vi "Select Sweep Mode.vi"(8 "error in (no error)":errorcluster, 10 "Sweep Modes":T1, 11 "NRT8000 in":refnum<class "NRT8000.lvclass">) -> (0 "error out":errorcluster, 3 "NRT8000 out":refnum<class "NRT8000.lvclass">)   [LabVIEW 2018, in "NRT8000.lvlib" / "NRT8000.lvclass"]
uses:
  NRT8000.lvclass
  PPLs/Optical Spectrum Analyzer/Parent/OSA.lvlibp/Custom Controls/enm_Sweep Modes.ctl
  PPLs/Optical Spectrum Analyzer/Parent/OSA.lvlibp/Optical Spectrum Analyzer.lvclass
  C:/Projects/LabVIEW/PPLs/Optical Spectrum Analyzer/Parent/OSA.lvlibp/Optical Spectrum Analyzer.lvclass
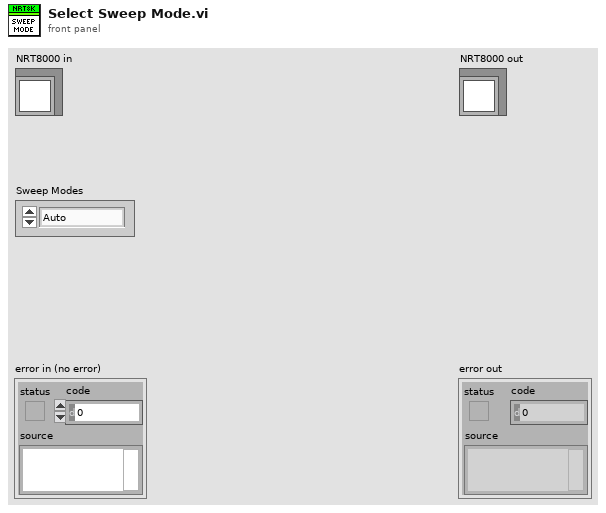
[diagram p1: front panel]
types:
  T1 = typedef "OSA.lvlibp/Optical Spectrum Analyzer.lvclass/enm_Sweep Modes.ctl" = enum16{"Auto", "Repeat", "Single", "Stop", "Segment"}
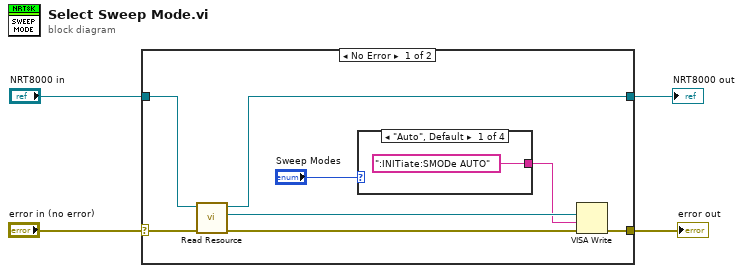
[diagram p0: block diagram]
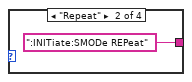
[diagram p2: hidden frame]
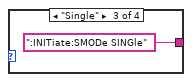
[diagram p3: hidden frame]
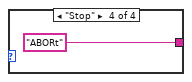
[diagram p4: hidden frame]
diagram:
  n1 = case shown="No Error" "error in (no error)" {
    selector: "error in (no error)" -> [w11 w18]
    tunnel: [w5 w18] -> w3
    tunnel: [w8 w17] -> w2
    tunnel: "NRT8000 in" -> [w9 w17]
    frame No Error {
      n2 = call "Read Resource.vi"("error in (no error)"=w11, "Optical Spectrum Analyzer in"=w9) -> ("error out"=w10:errorcluster, "Resource"=w7:refnum<visa-resource-name>, "Optical Spectrum Analyzer out"=w8:refnum<class "NRT8000.lvclass">)  [unwired: 7 in]
      n3 = case shown="\"Auto\", Default" "Sweep Modes" {
        tunnel: [":INITiate:SMODe AUTO" ":INITiate:SMODe REPeat" ":INITiate:SMODe SINGle" "ABORt"] -> w6
        frame "Auto", Default {
        }
        frame "Repeat" {
        }
        frame "Single" {
        }
        frame "Stop" {
        }
      }
      n4 = VISA Write(VISA resource name=w7, write buffer=w6, error in (no error)=w10) -> (error out=w5:errorcluster)  [unwired: 2 out]
    }
    frame Error {
    }
  }
  "error out" <- w3
  "NRT8000 out" <- w2
